vi "FGV_COM_PortHandler.vi"(4 "Device":T1, 5 "Error In":errorcluster, 7 "Action":T3) -> (0 "Error Out":errorcluster, 2 "Teaching Lab Arduinos":T2(array[cluster]), 3 "COM Port":refnum<visa-resource-name>)   [LabVIEW 2014]
uses:
  Typedef_FindPortActions.ctl
  Typedef_TeachLabArduinos.ctl
  <vilib>/regexp/Match Regular Expression.xnode
panel:
  out "Array":string[][](array[string])
  out "Current Check":refnum<visa-resource-name>
  out "Attempts Taken":i32[](array[numeric])
  out "COM only list":string[](array[string])
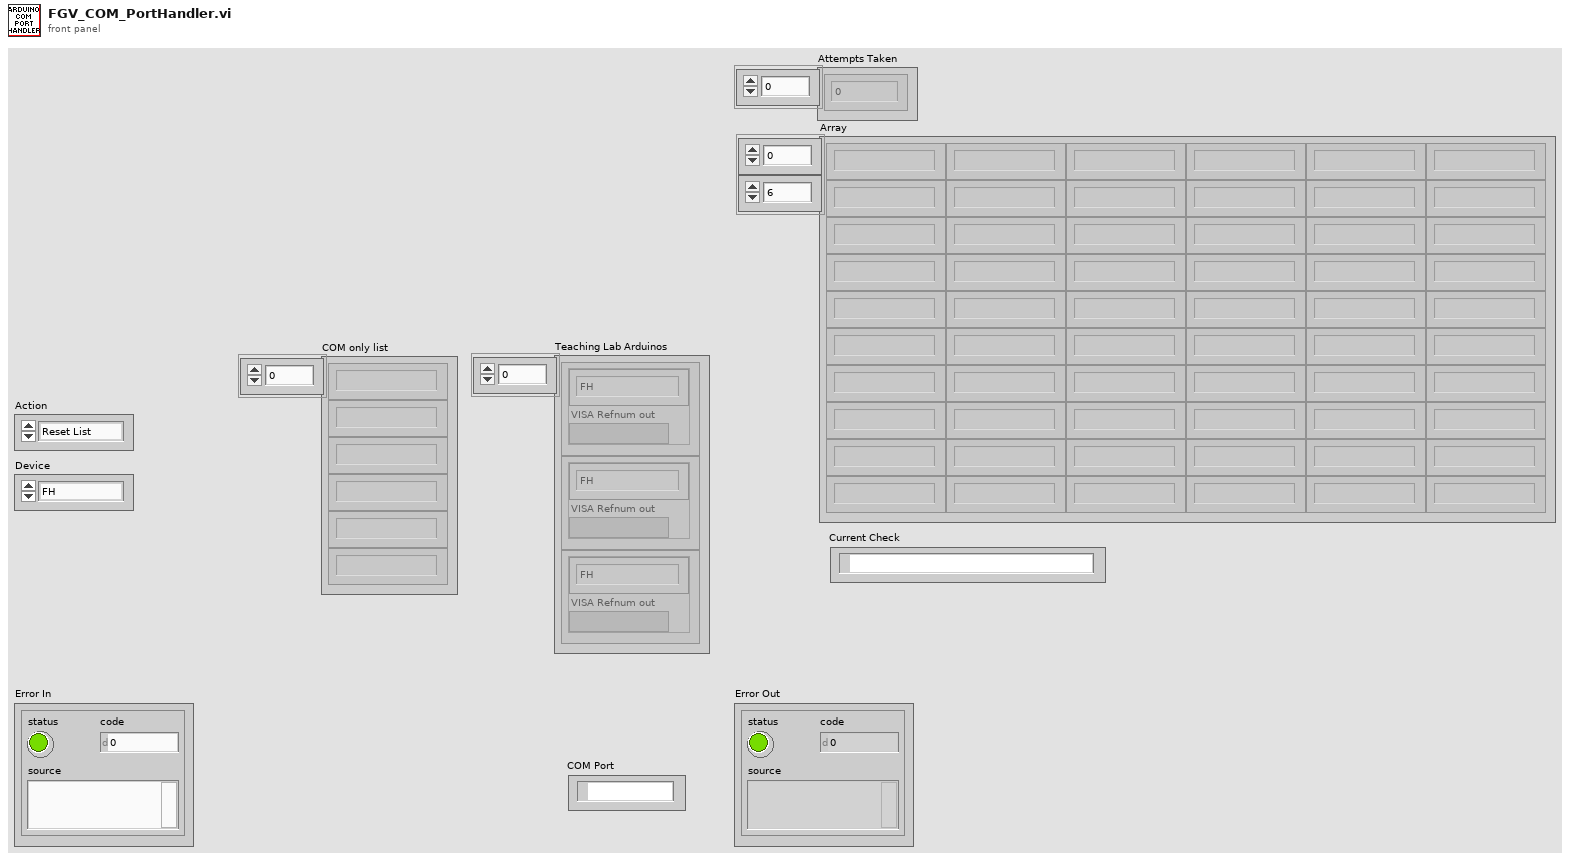
[diagram p1: front panel]
types:
  T1 = typedef "Typedef_TeachLabArduinos.ctl" = enum16{"FH", "AL", "CO", "TD"}
  T2 = cluster{T1, "VISA Refnum out":refnum<visa-resource-name>}[]
  T3 = typedef "Typedef_FindPortActions.ctl" = enum16{"Reset List", "Find arduinos", "Get COM Port"}
  T4 = cluster{T1, "VISA resource name out":refnum<visa-resource-name>}[]
  T5 = cluster{T1, "VISA Refnum out":refnum<visa-resource-name>}
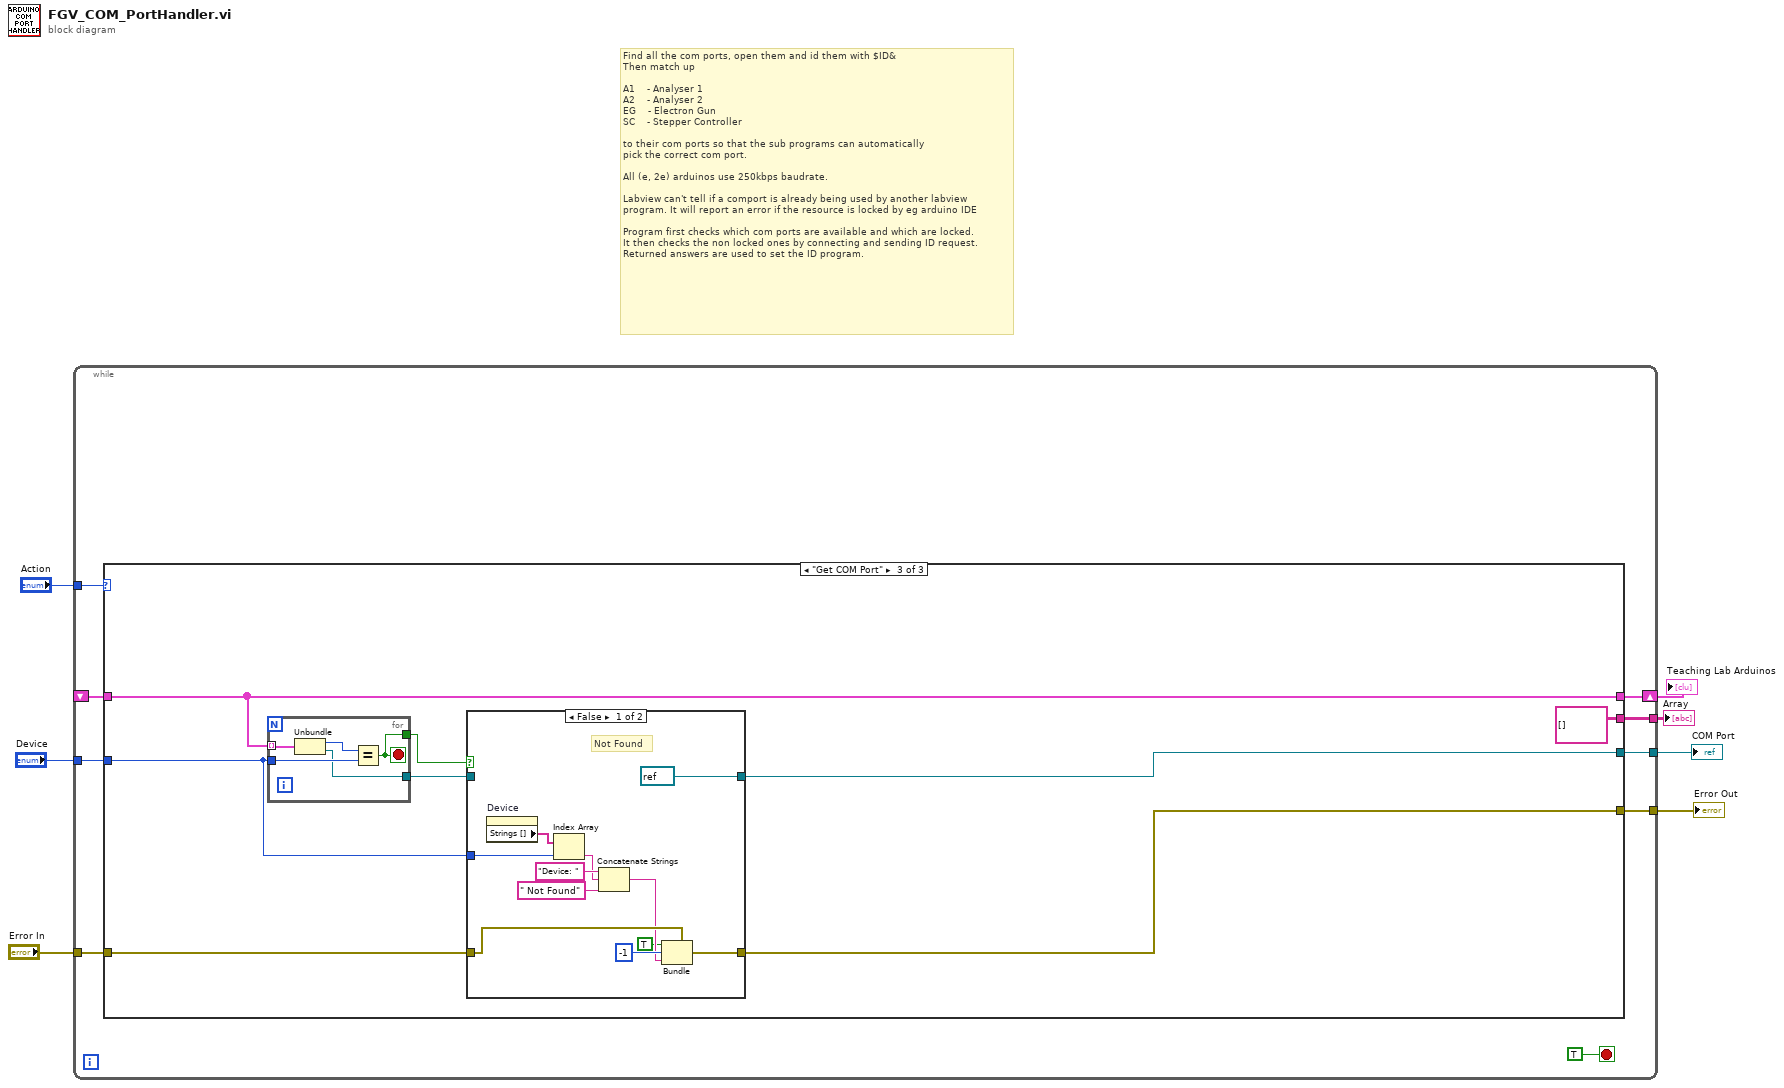
[diagram p0: block diagram]
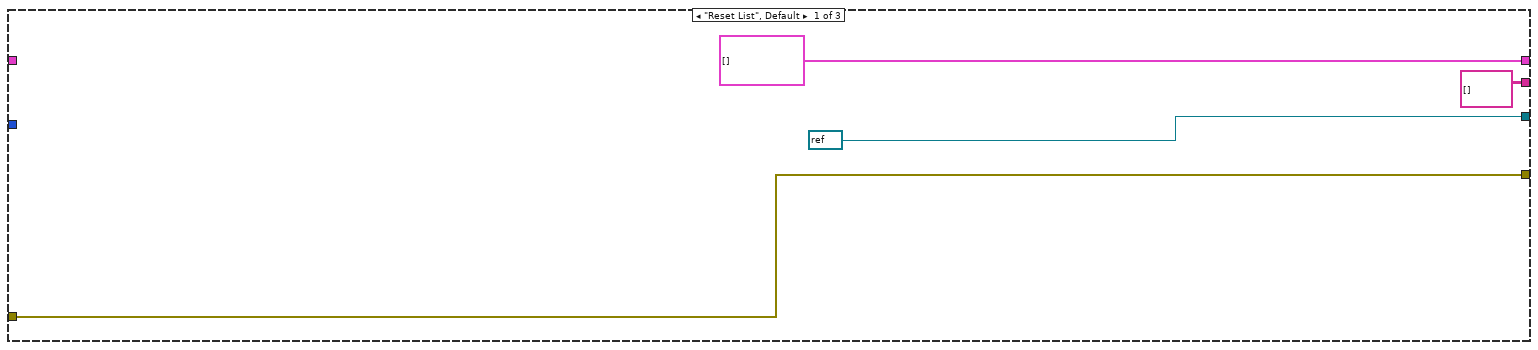
[diagram p2: hidden frame]
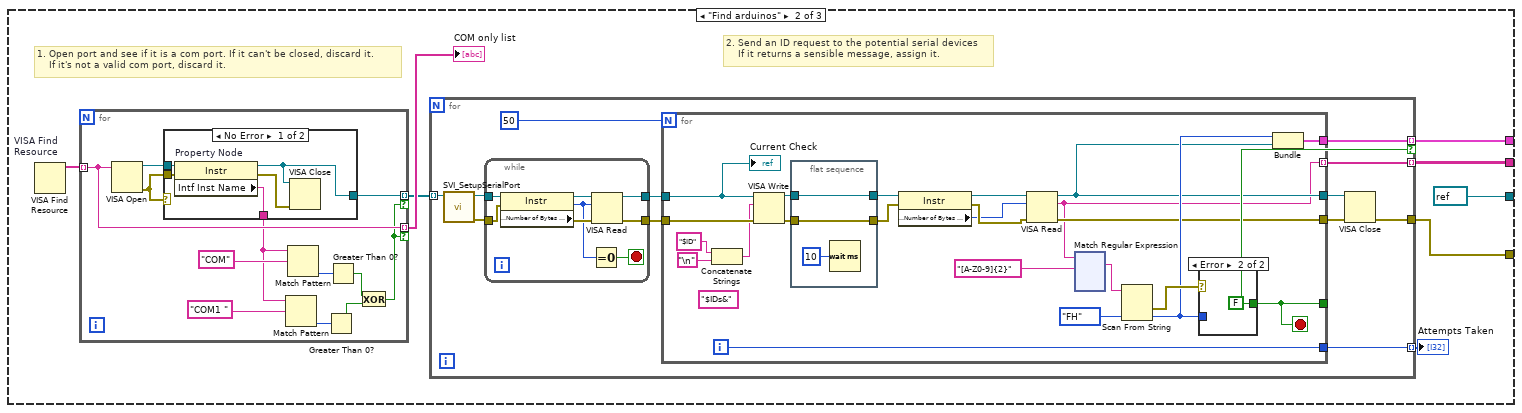
[diagram p3: hidden frame]
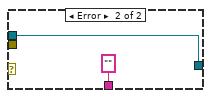
[diagram p4: hidden frame]
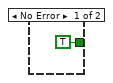
[diagram p5: hidden frame]
diagram:
  # "Find all the com ports, open them and id them with $ID&\nThen match up \n\nA1    - Analyser 1\nA2    - Analyser 2\nEG    - Electron Gun\nSC    - Stepper Controller\n\nto their com ports so that the sub programs can automatically\npick the correct com port.\n\nAll (e, 2e) arduinos use 250kbps baudrate.\n\nLabview can't tell if a comport is already being used by another labview\nprogram. It will report an error if the resource is locked by eg arduino IDE\n\nProgram first checks which com ports are available and which are locked.\nIt then checks the non locked ones by connecting and sending ID request.\nReturned answers are used to set the ID program."
  n1 = while {
    tunnel: "Action" -> [w15]
    shift-right: [w16] -> w1
    shift-left: _ -> [w13]
    tunnel: "Device" -> [w12]
    tunnel: [w11] -> w5
    tunnel: "Error In" -> [w10]
    tunnel: [w9] -> w4
    tunnel: [w8] -> w2
    stop <- TRUE stop-if-true
    n2 = case shown="\"Get COM Port\"" w15 {
      tunnel: [T4 [] w28 w218] -> w16
      tunnel: w13 -> [_ _ w218]
      tunnel: w12 -> [_ _ w212]
      tunnel: [refnum<visa-resource-name> refnum ("VISA resource name out") refnum<visa-resource-name> refnum ("VISA resource name out") w215] -> w11
      tunnel: w10 -> [w18 _ w211]
      tunnel: [w18 w23 w214] -> w9
      tunnel: [string[][] [] w21 string[][] []] -> w8
      frame "Reset List", Default {
      }
      frame "Find arduinos" {
        # "2. Send an ID request to the potential serial devices\n    If it returns a sensible message, assign it."
        # "1. Open port and see if it is a com port. If it can't be closed, discard it.\n    If it's not a valid com port, discard it."
        n3 = VISA Find Resource "VISA Find\nResource"() -> (3:w26:string[])  [unwired: 3 in, 2 out]
        n4 = for {
          tunnel: w26 -> [w37] mode=indexing
          tunnel: [w37] -> w25 mode=indexing if=w31
          tunnel: [w36] -> w24 mode=indexing if=w31
          n5 = VISA Open(VISA resource name=w37) -> (VISA resource name=w40:refnum<visa-resource-name>, error out=w29:errorcluster)  [unwired: 4 in]
          n6 = case shown="No Error" w29 {
            tunnel: w40 -> [w45 w47]
            tunnel: w29 -> [w44 _]
            tunnel: [w42 w47] -> w36
            tunnel: [w41 "" ("Intf Inst Name")] -> w30
            frame No Error {
              n7 = property on="Property Node" class="Instr"(reference=w45, error in=w44) -> (reference out=w42:refnum<visa-resource-name>, error out=w43:errorcluster, "Intf Inst Name"=w41:string)
              n8 = VISA Close(VISA resource name=w42, error in (no error)=w43) -> ()  [unwired: 1 out]
            }
            frame Error {
            }
          }
          n9 = Match Pattern(string=w30, regular expression="COM1 ") -> (offset past match=w35:i32)  [unwired: 1 in, 3 out]
          n10 = Match Pattern(string=w30, regular expression="COM") -> (offset past match=w38:i32)  [unwired: 1 in, 3 out]
          n11 = Greater Than 0?(x=w35) -> (x > 0?=w33:bool)
          n12 = Greater Than 0?(x=w38) -> (x > 0?=w32:bool)
          n13 = Exclusive Or(1:w33, 2:w32) -> (0:w31:bool)
        }
        "COM only list" <- w25
        n14 = for {
          tunnel: w24 -> [w55] mode=indexing
          tunnel: [w60] -> w28 mode=indexing if=w59
          tunnel: [w54] -> w23
          tunnel: [w53] -> w22 mode=indexing
          tunnel: [w52] -> w21 mode=indexing
          n15 = call "SVI_SetupSerialPort.vi"("VISA Refnum in"=w55) -> ("error out"=w50:errorcluster, "VISA Refnum out"=w49:refnum<visa-resource-name>)  [unwired: 9 in]
          n16 = while {
            tunnel: w49 -> [w64]
            tunnel: [w63] -> w48
            tunnel: w50 -> [w65]
            tunnel: [w66] -> w51
            stop <- w62 stop-if-true
            n17 = property class="Instr"(reference=w64, error in=w65) -> (reference out=w68:refnum<visa-resource-name>, error out=w67:errorcluster, "Serial Settings:Number of Bytes at Serial Port"=w61:u32)
            n18 = Equal To 0?(x=w61) -> (x = 0?=w62:bool)
            n19 = VISA Read(VISA resource name=w68, byte count=w61, error in (no error)=w67) -> (VISA resource name out=w63:refnum<visa-resource-name>, error out=w66:errorcluster)  [unwired: 2 out]
          }
          n20 = for {
            N: 50 -> [_]
            tunnel: w51 -> [w85]
            tunnel: w48 -> [w73]
            tunnel: [w80] -> w60
            tunnel: [w79] -> w59
            tunnel: [w78] -> w57
            tunnel: [w77] -> w56
            tunnel: [w74] -> w53
            tunnel: [w69] -> w52 mode=indexing
            i -> [w74]
            stop <- w79 stop-if-true
            (unwired) "$IDs&" ("write buffer")
            n21 = Concatenate Strings("$ID" ("write buffer"), "\n") -> (w70:string)
            n22 = VISA Write(VISA resource name=w73, write buffer=w70, error in (no error)=w85) -> (VISA resource name out=w87:refnum<visa-resource-name>, error out=w86:errorcluster)  [unwired: 1 out]
            n23 = flat-sequence {
              tunnel: [w209] -> w88
              tunnel: w87 -> [w209]
              tunnel: [w208] -> w89
              tunnel: w86 -> [w208]
              frame #0 {
                n24 = Wait (ms)(milliseconds to wait=u32 10) -> ()  [unwired: 1 out]
              }
            }
            n25 = property class="Instr"(reference=w88, error in=w89) -> (reference out=w91:refnum<visa-resource-name>, error out=w90:errorcluster, "Serial Settings:Number of Bytes at Serial Port"=w75:u32)
            n26 = VISA Read(VISA resource name=w91, byte count=w75, error in (no error)=w90) -> (VISA resource name out=w77:refnum<visa-resource-name>, read buffer=w69:string, error out=w78:errorcluster)  [unwired: 1 out]
            n27 = xnode "Match Regular Expression"("input string"=w69, "regular expression"="[A-Z0-9]{2}") -> ("whole match"=w76:string)  [unwired: 4 in, 4 out]
            n28 = Scan From String(input string=w76, default 1=Typedef_TeachLabArduinos."FH") -> (error out=w82:errorcluster, output 1=w81:T1)  [unwired: 3 in, 2 out]
            n29 = case shown="Error" w82 {
              tunnel: w81 -> [_ _]
              tunnel: [TRUE FALSE] -> w79
              frame No Error {
              }
              frame Error {
              }
            }
            n30 = Bundle(w81, "VISA Refnum out"=w77) -> (w80:T5)  [unwired: 1 in]
            "Current Check" <- w73
          }
          n31 = VISA Close(VISA resource name=w56, error in (no error)=w57) -> (error out=w54:errorcluster)
        }
        "Attempts Taken" <- w22
      }
      frame "Get COM Port" {
        n32 = for {
          tunnel: w218 -> [w236] mode=indexing
          tunnel: w212 -> [w235]
          tunnel: [w233] -> w216
          tunnel: [w232] -> w217
          stop <- w232 stop-if-true
          n33 = Unbundle(w236) -> (w234:T1, "VISA Refnum out"=w233:refnum<visa-resource-name>)
          n34 = Equal?(x=w234, y=w235) -> (x = y?=w232:bool)
        }
        n35 = case shown="False" w217 {
          tunnel: [refnum<visa-resource-name> refnum ("VISA resource name out") w231] -> w215
          tunnel: w216 -> [_ w231]
          tunnel: w211 -> [w222 w230]
          tunnel: [w223 w230] -> w214
          tunnel: w212 -> [w225 _]
          frame False {
            # "Not Found"
            n36 = property on="Device" class="Enum (strict)"() -> ("Strings []"=w226:string[])  [unwired: 2 in, 2 out]
            n37 = Index Array(array=w226, index=w225) -> (element=w224:string)
            n38 = Concatenate Strings("Device: " ("string"), w224, " Not Found" ("String to Prepend to source (\"\")")) -> (w220:string)
            n39 = Bundle(cluster=w222, "status"=TRUE, "code"=-1, "source"=w220) -> (w223:errorcluster)
          }
          frame True {
            # "Found"
          }
        }
      }
    }
  }
  "COM Port" <- w5
  "Error Out" <- w4
  "Array" <- w2
  "Teaching Lab Arduinos" <- w1
